vi "method_redraw.vi"(0 "Display State In":T1={"current frame index"=0, "number of images"=0, "ROI (frames)"={"ROI"=[]}, "control refs"={"frame"=refnum, "image"=refnum, "saveROIsButton"=refnum, "loadImageSwitch"=refnum, "loadROIsSwitch"=refnum, "saveROIsSwitch"=refnum, "loadImagePath"=refnum, "loadROIPath"=refnum, "redraw"=refnum}, "calibration"={"x"=0.0, "y"=0.0, "x unit"=enum."um", "y unit"=enum."um"}, "xpaths"={"x offset"="", "y offset"="", "z offset"=""}, "offset"=refnum, "XML description"="", "number of ROIs"=0.0, "ROI Tool Buttons Visible"={"Zoom Tool"=FALSE, "Selection Tool"=FALSE, "Pan Tool"=FALSE, "Point Tool"=FALSE, "Line Tool"=FALSE, "Rectangle Tool"=FALSE, "Rotated Rectangle Tool"=FALSE, "Polyline Tool"=FALSE, "Polygon Tool"=FALSE, "Freehand Tool"=FALSE, "Closed Freehand Tool"=FALSE, "Ellipse Tool"=FALSE, "Annulus Tool"=FALSE}, "ROI color"=0, "number color"=0, "enable ROI numbering?"=FALSE, "selected path to save ROIs"=path "", "starting path"=path "", "array of overlays"=[], "pointCollection"=refnum, "ROImode"=enum."IMAQROIs", "selected point ID"=0.0, "point radius"=5, "point colours"=[], "PlotAreaSize"={"Width"=0, "Height"=0}, "last action"=enum."not specified"} {"array of overlays"."overlay size" min=1}, 9 "Container State":T10, 11 "error in (no error)":errorcluster) -> (4 "Display State Out":T1={"current frame index"=0, "number of images"=0, "ROI (frames)"={"ROI"=[]}, "control refs"={"frame"=refnum, "image"=refnum, "saveROIsButton"=refnum, "loadImageSwitch"=refnum, "loadROIsSwitch"=refnum, "saveROIsSwitch"=refnum, "loadImagePath"=refnum, "loadROIPath"=refnum, "redraw"=refnum}, "calibration"={"x"=0.0, "y"=0.0, "x unit"=enum."um", "y unit"=enum."um"}, "xpaths"={"x offset"="", "y offset"="", "z offset"=""}, "offset"=refnum, "XML description"="", "number of ROIs"=0.0, "ROI Tool Buttons Visible"={"Zoom Tool"=FALSE, "Selection Tool"=FALSE, "Pan Tool"=FALSE, "Point Tool"=FALSE, "Line Tool"=FALSE, "Rectangle Tool"=FALSE, "Rotated Rectangle Tool"=FALSE, "Polyline Tool"=FALSE, "Polygon Tool"=FALSE, "Freehand Tool"=FALSE, "Closed Freehand Tool"=FALSE, "Ellipse Tool"=FALSE, "Annulus Tool"=FALSE}, "ROI color"=0, "number color"=0, "enable ROI numbering?"=FALSE, "selected path to save ROIs"=path "", "starting path"=path "", "array of overlays"=[], "pointCollection"=refnum, "ROImode"=enum."IMAQROIs", "selected point ID"=0.0, "point radius"=5, "point colours"=[], "PlotAreaSize"={"Width"=0, "Height"=0}, "last action"=enum."not specified"} {"array of overlays"."overlay size" min=1}, 15 "error out":errorcluster)   [LabVIEW 2010, in "XImage.xctl"]
uses:
  XImage.xctl
  <vilib>/_xctls/Container State.ctl
  state.ctl
  classes/SpaceVector/SpaceVector/SpaceVector.lvclass
  classes/PointCollection/PointCollection/PointCollection.lvclass
  ROI_frames_cluster.ctl
  control_refs_cluster.ctl
  calibration_cluster.ctl
  enumerations/unit.ctl
  xpath_cluster.ctl
  overlays_cluster.ctl
  ROI_mode_enum.ctl
  last_action_enum.ctl
  <vilib>/_xctls/XControlSupport.lvlib
  classes/Image/Image/Image.lvclass
panel:
  # "Add Controls & Indicators that form the parameters of the method here. Hook them to the connector pane. Do not delete the controls & indicators that are already hooked to the connector pane.\n \nTo setup the parameters  for this method, right click on this item in the Project Tree & select \"Configure Method...\"."
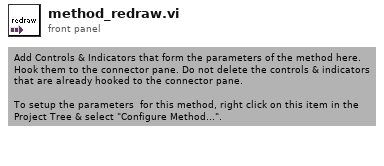
[diagram p1: front panel]
types:
  T1 = typedef "XImage.xctl/state.ctl" = cluster{"current frame index":i32, "number of images":i32, "ROI (frames)":T2, "control refs":T3, "calibration":T4, "xpaths":T6, "offset":refnum<class "SpaceVector.lvclass">, "XML description":string, "number of ROIs":dbl, "ROI Tool Buttons Visible":cluster{"Zoom Tool":bool, "Selection Tool":bool, "Pan Tool":bool, "Point Tool":bool, "Line Tool":bool, "Rectangle Tool":bool, "Rotated Rectangle Tool":bool, "Polyline Tool":bool, "Polygon Tool":bool, "Freehand Tool":bool, "Closed Freehand Tool":bool, "Ellipse Tool":bool, "Annulus Tool":bool}, "ROI color":u32, "number color":u32, "enable ROI numbering?":bool, "selected path to save ROIs":path, "starting path":path, "array of overlays":T7[], "pointCollection":refnum<class "PointCollection.lvclass">, "ROImode":T8, "selected point ID":dbl, "point radius":i32, "point colours":u32[], "PlotAreaSize":cluster{"Width":u32, "Height":u32}, "last action":T9}
  T2 = typedef "XImage.xctl/ROI_frames_cluster.ctl" = cluster{"ROI":cluster{"Global Rectangle":i32[], "Contours":cluster{"Contour Type":u32, "ROI Type":u32, "Points":i32[]}[]}[]}
  T3 = typedef "XImage.xctl/control_refs_cluster.ctl" = cluster{"frame":refnum<vi>, "image":refnum<vi>, "saveROIsButton":refnum<vi>, "loadImageSwitch":refnum<vi>, "loadROIsSwitch":refnum<vi>, "saveROIsSwitch":refnum<vi>, "loadImagePath":refnum<vi>, "loadROIPath":refnum<vi>, "redraw":refnum<vi>}
  T4 = typedef "XImage.xctl/calibration_cluster.ctl" = cluster{"x":dbl, "y":dbl, "x unit":T5, "y unit":T5}
  T5 = typedef "Image.lvclass/unit.ctl" = enum16{"um", "s"}
  T6 = typedef "XImage.xctl/xpath_cluster.ctl" = cluster{"x offset":string, "y offset":string, "z offset":string}
  T7 = typedef "XImage.xctl/overlays_cluster.ctl" = cluster{"overlay array":cluster{i32[][]}[], "overlay name":string, "color (red)":u32, "overlay size":i32, "overlay type":enum16{"crosshair", "circle"}}
  T8 = typedef "XImage.xctl/ROI_mode_enum.ctl" = enum16{"none", "IMAQROIs", "PointCollection"}
  T9 = typedef "XImage.xctl/last_action_enum.ctl" = enum16{"not specified", "image loaded", "frame changed", "ROIs changed"}
  T10 = typedef "XControlSupport.lvlib/Container State.ctl" = cluster{"Indicator?":bool, "Run Mode?":bool, " Refnum":refnum<vi>}
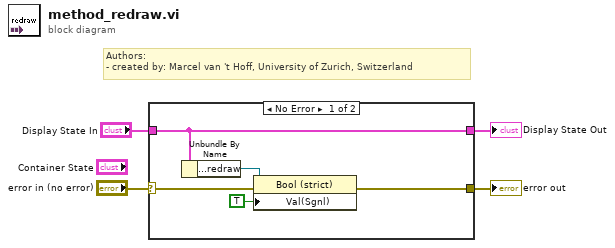
[diagram p0: block diagram]
diagram:
  # "Authors: \n- created by: Marcel van 't Hoff, University of Zurich, Switzerland"
  n1 = case shown="No Error" "error in (no error)" {
    selector: "error in (no error)" -> [w7 w11]
    tunnel: "Display State In" -> [w6 w10]
    tunnel: [w5 w11] -> w3
    tunnel: [w6 w10] -> w1
    frame No Error {
      n2 = Unbundle By Name(w6) -> ("control refs.redraw"=w9:refnum<vi>)
      n3 = property class="Bool (strict)"(reference=w9, error in=w7, "Val(Sgnl)"=TRUE ("Value")) -> (error out=w5:errorcluster)  [unwired: 1 out]
    }
    frame Error {
    }
  }
  "Display State Out" <- w1
  "error out" <- w3
